vi "coerce width height.vi"(8 "Offset Y":i64(slide) min=0 max=1196 step=4 scale=0.0..1196.0, 11 "Offset X":i64(slide) min=0 max=1916 step=4 scale=0.0..1916.0) -> (0 "max height":i64=1200, 3 "max width":i64=1920)   [LabVIEW 2020]
panel:
  # "given x and y offsets, calc the max width and height. coerce later"
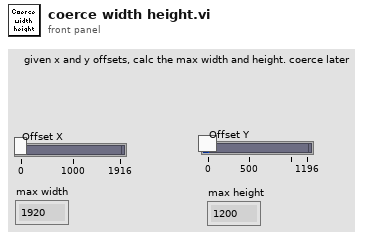
[diagram p1: front panel]
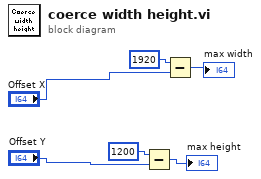
[diagram p0: block diagram]
diagram:
  n1 = Subtract(x=1200, y="Offset Y") -> (x-y=→"max height":i64)
  n2 = Subtract(x=1920, y="Offset X") -> (x-y=→"max width":i64)
